vi "calculate_extinction_angle_with_tilt_correction.vi"(8 "Error In":errorcluster, 11 "Xtal Description":T1) -> (0 "Error Out":errorcluster, 3 "prediction":dbl)   [LabVIEW 2019]
doc: "Calculate the predicted extinction angle with the tilt correction - all I/O in radians. Based on the old code."
uses:
  xtal_description_for_prediction_cluster_typedef.ctl
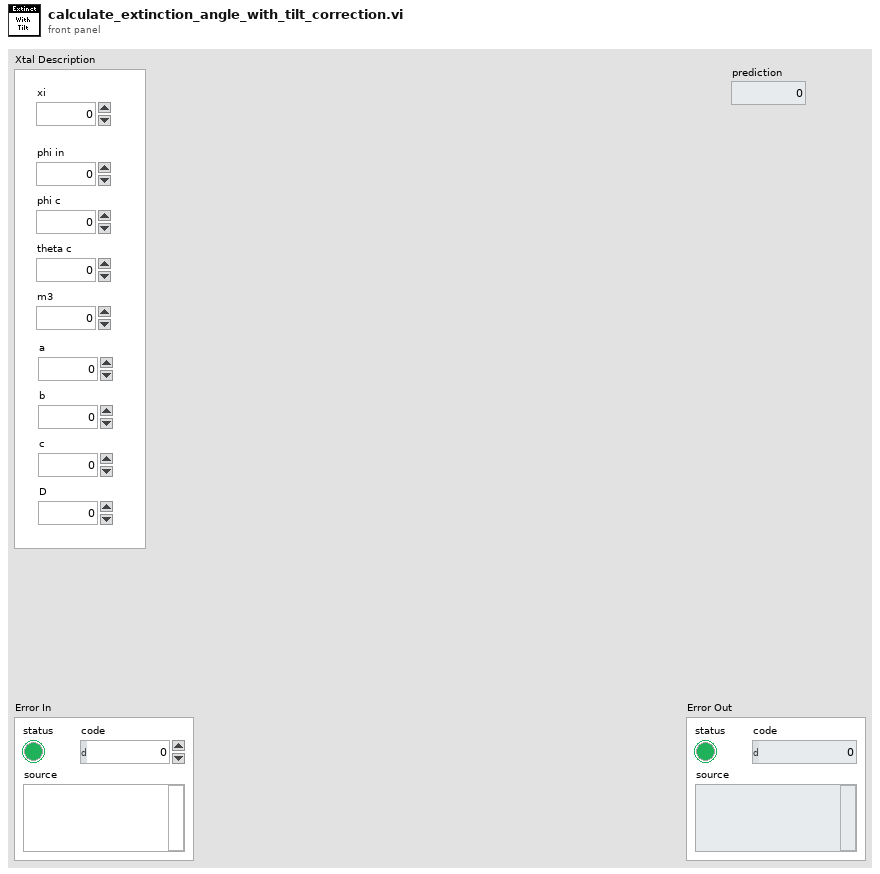
[diagram p1: front panel]
types:
  T1 = typedef "xtal_description_for_prediction_cluster_typedef.ctl" = cluster{"xi":dbl, "phi in":dbl, "phi c":dbl, "theta c":dbl, "m3":dbl, "a":dbl, "b":dbl, "c":dbl, "D":dbl}
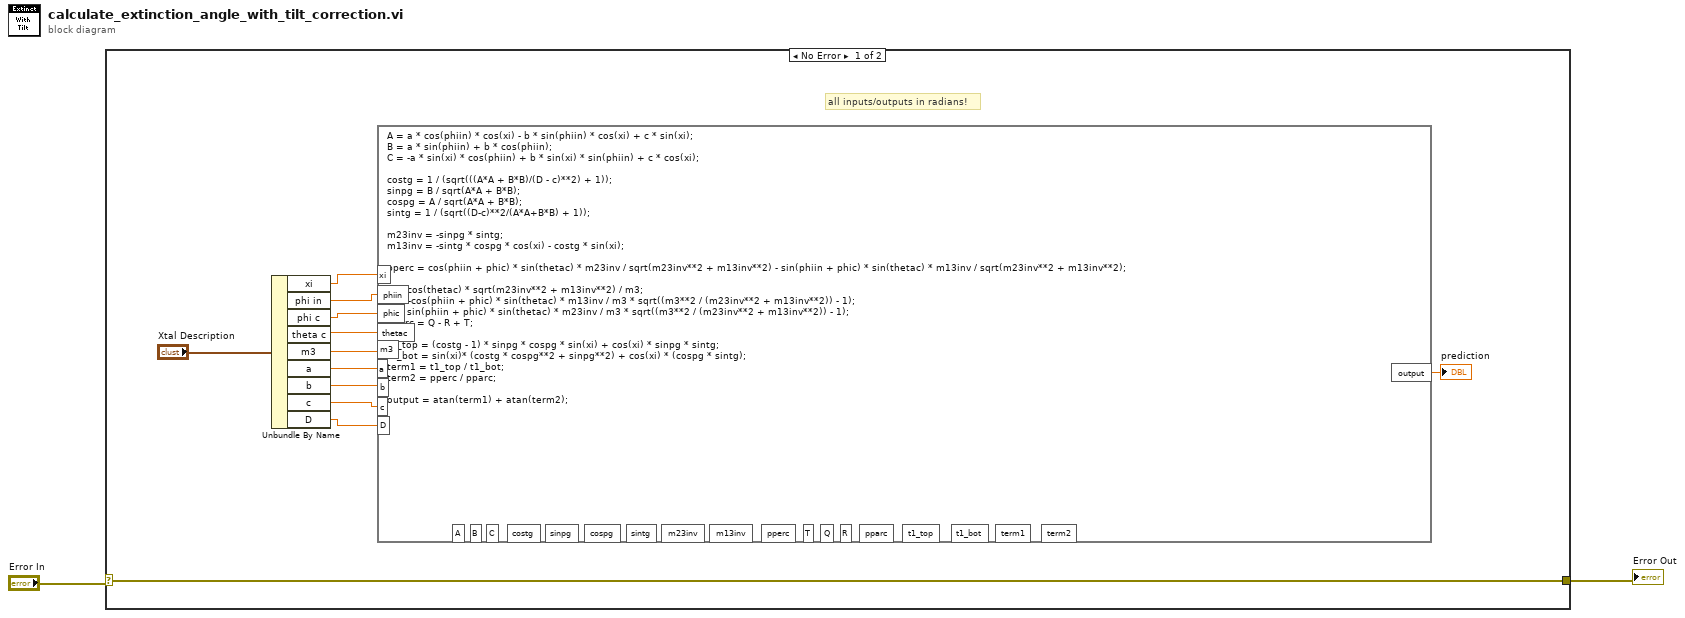
[diagram p0: block diagram]
diagram:
  n1 = case shown="No Error" "Error In" {
    selector: "Error In" -> [w3 w15]
    tunnel: [w3 w15] -> w1
    frame No Error {
      # "all inputs/outputs in radians!"
      n2 = Unbundle By Name("Xtal Description") -> ("xi"=w13:dbl, "phi in"=w12:dbl, "phi c"=w11:dbl, "theta c"=w10:dbl, "m3"=w9:dbl, "a"=w8:dbl, "b"=w7:dbl, "c"=w6:dbl, "D"=w5:dbl)
      n3 = formula code="A = a * cos(phiin) * cos(xi) - b * sin(phiin) * cos(xi) + c * sin(xi);\nB = a * sin(phiin) + b * cos(phiin);\nC = -a * sin(xi) * cos(phiin) + b * sin(xi) * sin(phiin) + c * cos(xi);\n\ncostg = 1 / (sqrt(((A*A + B*B)/(D - c)**2) + 1));\nsinpg = B / sqrt(A*A + B*B);\ncospg = A / sqrt(A*A + B*B);\nsintg = 1 / (sqrt((D-c)**2/(A*A+B*B) + 1));\n\nm23inv = -sinpg * sintg;\nm13inv = -sintg * cospg * cos(xi) - costg * sin(xi);\n\npperc = cos(phiin + phic) * sin(thetac) * m23inv / sqrt(m23inv**2 + m13inv**2) - sin(phiin + phic) * sin(thetac) * m13inv / sqrt(m23inv**2 + m13inv**2);\n\nT = cos(thetac) * sqrt(m23inv**2 + m13inv**2) / m3;\nQ = -cos(phiin + phic) * sin(thetac) * m13inv / m3 * sqrt((m3**2 / (m23inv**2 + m13inv**2)) - 1);\nR = sin(phiin + phic) * sin(thetac) * m23inv / m3 * sqrt((m3**2 / (m23inv**2 + m13inv**2)) - 1);\npparc = Q - R + T;\n\nt1_top = (costg - 1) * sinpg * cospg * sin(xi) + cos(xi) * sinpg * sintg;\nt1_bot = sin(xi)* (costg * cospg**2 + sinpg**2) + cos(xi) * (cospg * sintg);\nterm1 = t1_top / t1_bot;\nterm2 = pperc / pparc;\n\noutput = atan(term1) + atan(term2);"("xi"=w13, "phiin"=w12, "phic"=w11, "thetac"=w10, "m3"=w9, "a"=w8, "b"=w7, "c"=w6, "D"=w5) -> ("output"=→"prediction":dbl)  [unwired: 18 out]
    }
    frame Error {
    }
  }
  "Error Out" <- w1
